vi "prepare function list.vi"(5 "sort?":bool, 6 "error in":errorcluster, 8 "Functions listbox":refnum<vi>, 9 "configuration in":refnum<class "fixed channel tag bus module configuration.lvclass">) -> (0 "error out":errorcluster, 3 "configuration out":refnum<class "fixed channel tag bus module configuration.lvclass">)   [LabVIEW 2013]
uses:
  module/configuration/fixed channel tag bus module configuration.lvclass
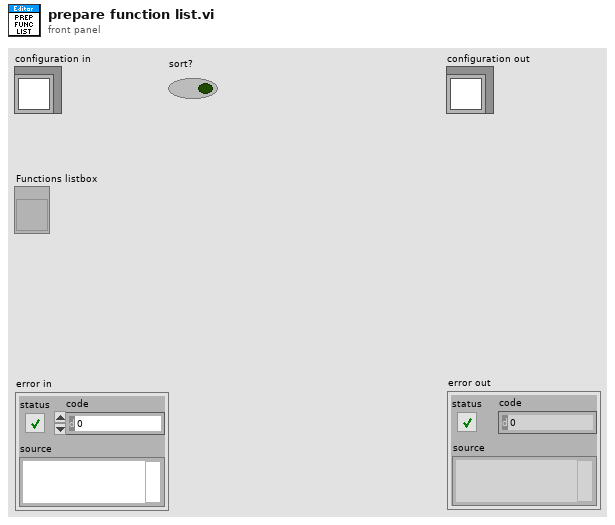
[diagram p1: front panel]
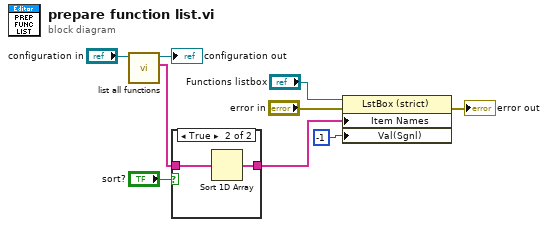
[diagram p0: block diagram]
diagram:
  n1 = call "list all functions.vi"("user module configuration in"="configuration in") -> ("functions"=w1:string[], "user module configuration out"=→"configuration out":refnum<class "test 4 configuration.lvclass">)  [unwired: 9 in]
  n2 = case shown="True" "sort?" {
    tunnel: [w10 w11] -> w2
    tunnel: w1 -> [w10 w12]
    frame False {
    }
    frame True {
      n3 = Sort 1D Array(array=w12) -> (sorted array=w11:string[])
    }
  }
  n4 = property class="LstBox (strict)"(reference="Functions listbox", error in="error in", "Item Names"=w2, "Val(Sgnl)"=-1 ("Value (Signaling)")) -> (error out=→"error out":errorcluster)  [unwired: 1 out]
